vi "Test VI Debugging Disabled.vi"(8 "error in (no error)":errorcluster, 10 "VI Refnum":refnum<vi>, 11 "TestCase in":refnum<class "TestCase.lvclass">) -> (0 "error out":errorcluster, 3 "TestCase out":refnum<class "TestCase.lvclass">)   [LabVIEW 2011]
doc: "Test for VI is reentrant and has the reentrancy type specified."
uses:
  <vilib>/addons/_JKI Toolkits/VI Tester/TestCase.llb/TestCase.lvclass
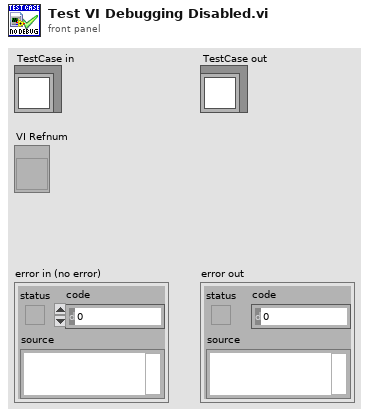
[diagram p1: front panel]
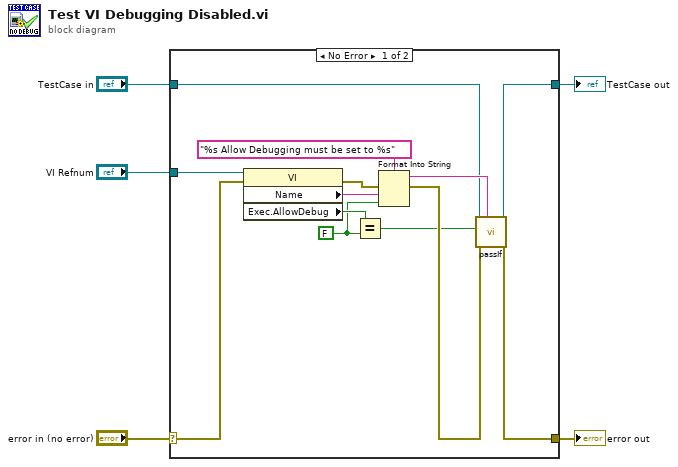
[diagram p0: block diagram]
diagram:
  n1 = case shown="No Error" "error in (no error)" {
    selector: "error in (no error)" -> [w10 w19]
    tunnel: [w16 w19] -> w5
    tunnel: "TestCase in" -> [w15 w20]
    tunnel: [w14 w20] -> w3
    tunnel: "VI Refnum" -> [w13 _]
    frame No Error {
      w7 = FALSE
      n2 = property class="VI"(reference=w13, error in=w10) -> (error out=w12:errorcluster, "Name"=w9:string, "Exec.AllowDebug"=w8:bool)  [unwired: 1 out]
      n3 = Equal?(x=w8, y=w7) -> (x = y?=w6:bool)
      n4 = Format Into String(format string="%s Allow Debugging must be set to %s" ("custom report message (\"\")"), error in=w12, w9, w7) -> (resulting string=w17:string, error out=w11:errorcluster)  [unwired: 1 in]
      n5 = call-dynamic "passIf.vi"("custom report message (\"\")"=w17, "error in (no error)"=w11, "pass"=w6, "TestCase in"=w15) -> ("error out"=w16:errorcluster, "TestCase out"=w14:refnum<class "TestCase.lvclass">)  [unwired: 6 in]
    }
    frame Error {
    }
  }
  "error out" <- w5
  "TestCase out" <- w3
